vi "img test.vi"() -> ()   [LabVIEW 2009]
uses:
  <vilib>/vision/NI_Vision_Development_Module.lvlib
panel:
  in  "Operation 1":T1(ring)=enum."Erode"
  out "Image 4":T2(plugin-control)
  out "Image 3":T2(plugin-control)
  in  "Color Plane":i32(ring)=1 items=["Red", "Green", "Blue", "Hue", "Saturation", "Luminance", "Value", "Intensity"]
  in  "Structuring Element":i32[][](array[numeric])=[[1, 1, 1]]
  in  "startign rame":i32
  in  "Number of iterations (1)":i32=1
  in  "frame diff":i32
  out "Image 2":T2(plugin-control)
  in  "Range 2":cluster{"Lower value":sgl, "Upper value":sgl}={"Lower value"=128.0, "Upper value"=255.0} {"Upper value" format="%.2f"; "Lower value" format="%.2f"}
  in  "stop":bool
  in  "Range":cluster{"Lower value":sgl, "Upper value":sgl}={"Lower value"=128.0, "Upper value"=255.0} {"Upper value" format="%.2f"; "Lower value" format="%.2f"}
  out "Image":T2(plugin-control)
  in  "AVI Path":path=path "C:/Users/Kokum Weeratunga/Desktop/ChongWei vs LinDan (japan open 2010).avi"
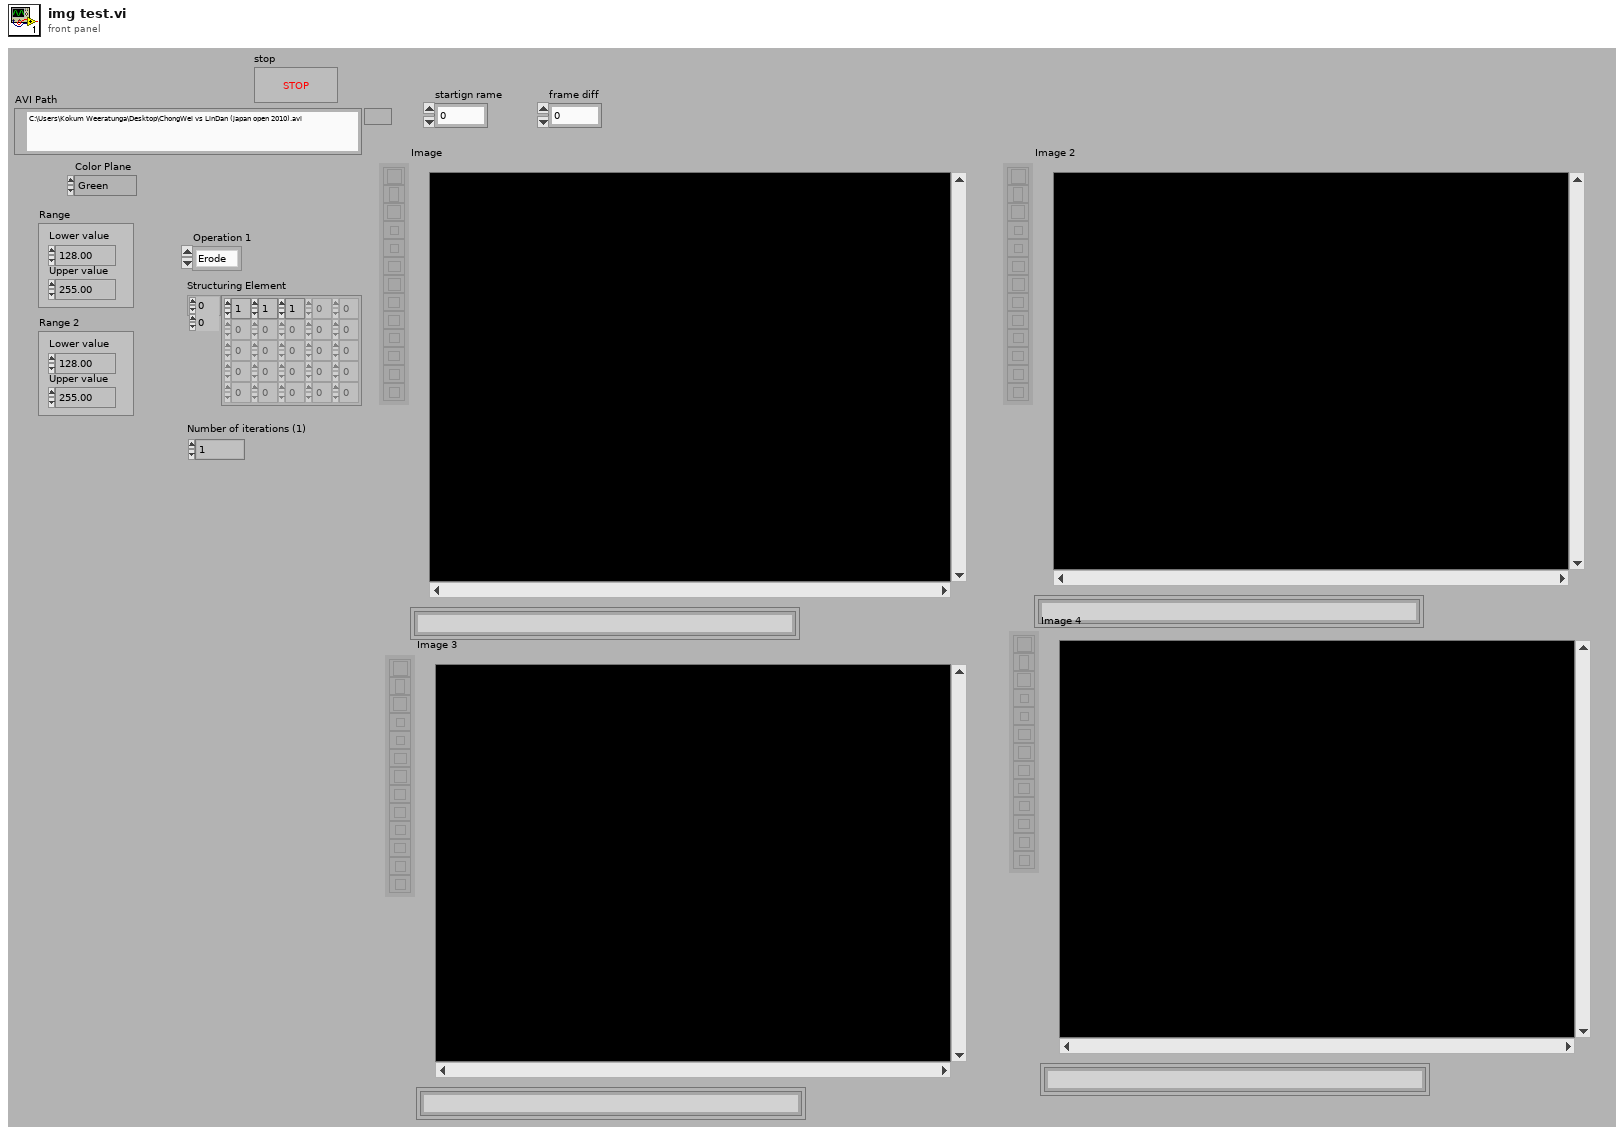
[diagram p1: front panel]
types:
  T1 = enum32{"AutoM", "Close", "Dilate", "Erode", "Gradient", "Gradient in", "Gradient out", "HitMiss", "Open", "PClose", "POpen", "Thick", "Thin"}
  T2 = typedef "IMAQ Image.ctl" = refnum<image>
  T3 = typedef "Image Type" = u32
  T4 = typedef "AviRefnum.ctl" = refnum<k1>
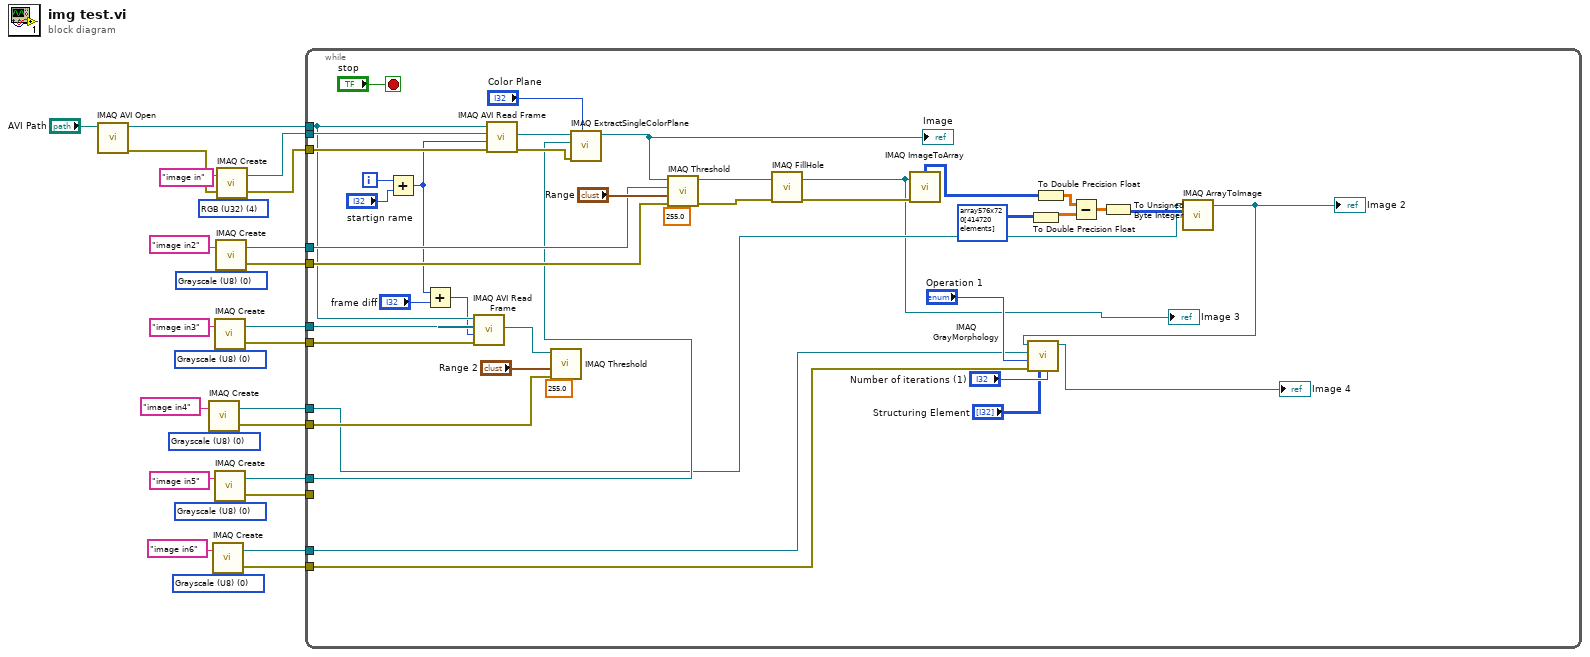
[diagram p0: block diagram]
diagram:
  w3 = T3 0 items=["Grayscale (U8)", "Grayscale (I16)", "Grayscale (SGL)", "Complex (CSG)", "RGB (U32)", "HSL (U32)", "RGB (U64)", "Grayscale (U16)"] ("Image Type")
  w14 = T3 0 items=["Grayscale (U8)", "Grayscale (I16)", "Grayscale (SGL)", "Complex (CSG)", "RGB (U32)", "HSL (U32)", "RGB (U64)", "Grayscale (U16)"] ("Image Type")
  w12 = T3 0 items=["Grayscale (U8)", "Grayscale (I16)", "Grayscale (SGL)", "Complex (CSG)", "RGB (U32)", "HSL (U32)", "RGB (U64)", "Grayscale (U16)"] ("Image Type")
  w16 = T3 0 items=["Grayscale (U8)", "Grayscale (I16)", "Grayscale (SGL)", "Complex (CSG)", "RGB (U32)", "HSL (U32)", "RGB (U64)", "Grayscale (U16)"] ("Image Type")
  w19 = T3 0 items=["Grayscale (U8)", "Grayscale (I16)", "Grayscale (SGL)", "Complex (CSG)", "RGB (U32)", "HSL (U32)", "RGB (U64)", "Grayscale (U16)"] ("Image Type")
  w22 = T3 4 items=["Grayscale (U8)", "Grayscale (I16)", "Grayscale (SGL)", "Complex (CSG)", "RGB (U32)", "HSL (U32)", "RGB (U64)", "Grayscale (U16)"] ("Image Type")
  n1 = call "IMAQ AVI Open"("AVI Path"="AVI Path") -> ("error out"=w26:errorcluster, "Avi Refnum"=w21:T4)  [unwired: 9 in]
  n2 = call "IMAQ Create"("Image Name"="image in4", "Image Type"=w14) -> ("New Image"=w8:T2, "error out"=w7:errorcluster)  [unwired: 3 in]
  n3 = call "IMAQ Create"("Image Name"="image in6", "Image Type"=w3) -> ("New Image"=w2:T2, "error out"=w1:errorcluster)  [unwired: 3 in]
  n4 = call "IMAQ Create"("Image Name"="image in3", "Image Type"=w12) -> ("New Image"=w10:T2, "error out"=w9:errorcluster)  [unwired: 3 in]
  n5 = call "IMAQ Create"("Image Name"="image in5", "Image Type"=w16) -> ("New Image"=w6:T2, "error out"=w5:errorcluster)  [unwired: 3 in]
  n6 = call "IMAQ Create"("Image Name"="image in2", "Image Type"=w19) -> ("New Image"=w18:T2, "error out"=w17:errorcluster)  [unwired: 3 in]
  n7 = call "IMAQ Create"("Image Name"="image in", "Image Type"=w22, "error in (no error)"=w26) -> ("New Image"=w23:T2, "error out"=w24:errorcluster)  [unwired: 2 in]
  n8 = while {
    tunnel: w24 -> [w69]
    tunnel: w23 -> [w68]
    tunnel: w21 -> [w59]
    tunnel: w18 -> [w65]
    tunnel: w17 -> [w64]
    tunnel: w10 -> [w58]
    tunnel: w9 -> [w57]
    tunnel: w8 -> [w33]
    tunnel: w7 -> [w42]
    tunnel: w6 -> [w43]
    tunnel: w5 -> [_]
    tunnel: w2 -> [w29]
    tunnel: w1 -> [w55]
    i -> [w52]
    stop <- "stop" stop-if-true
    n9 = Add(x=w52, y="startign rame") -> (x+y=w49:i32)
    n10 = Add(x=w49, y="frame diff") -> (x+y=w56:i32)
    n11 = call "IMAQ AVI Read Frame"("error in (no error)"=w57, "Frame Number"=w56, "Image"=w58, "Avi Refnum"=w59) -> ("Image Out"=w62:T2)  [unwired: 4 in, 3 out]
    n12 = call "IMAQ AVI Read Frame"("error in (no error)"=w69, "Frame Number"=w49, "Image"=w68, "Avi Refnum"=w59) -> ("error out"=w46:errorcluster, "Image Out"=w47:T2)  [unwired: 4 in, 2 out]
    n13 = call "IMAQ Threshold"("Replace Value"=sgl 255.0, "error in (no error)"=w42, "Range"="Range 2", "Image Src"=w62) -> ()  [unwired: 6 in, 2 out]
    n14 = call "IMAQ ExtractSingleColorPlane"("Color Plane"="Color Plane", "error in (no error)"=w46, "Image Dst"=w43, "Image Src"=w47) -> ("Image Dst Out"=w44:T2)  [unwired: 6 in, 1 out]
    "Image" <- w44
    n15 = call "IMAQ Threshold"("Replace Value"=sgl 255.0, "error in (no error)"=w64, "Range"="Range", "Image Dst"=w65, "Image Src"=w44) -> ("error out"=w40:errorcluster, "Image Dst Out"=w41:T2)  [unwired: 5 in]
    n16 = call "IMAQ FillHole"("error in (no error)"=w40, "Image Src"=w41) -> ("error out"=w36:errorcluster, "Image Dst Out"=w32:T2)  [unwired: 4 in]
    "Image 3" <- w32
    n17 = call "IMAQ ImageToArray"("error in (no error)"=w36, "Image"=w32) -> ("Image Pixels (U8)"=w35:u8[][])  [unwired: 2 in, 4 out]
    n18 = To Double Precision Float(number=u8[][] array576x720[414720 elements] ("Image Pixels (U8)")) -> (double precision float=w37:dbl[][])
    n19 = To Double Precision Float(number=w35) -> (double precision float=w38:dbl[][])
    n20 = Subtract(x=w38, y=w37) -> (x-y=w39:dbl[][])
    n21 = To Unsigned Byte Integer(number=w39) -> (unsigned 8bit integer=w34:u8[][])
    n22 = call "IMAQ ArrayToImage"("Image Pixels (U8)"=w34, "Image"=w33) -> ("Image Out"=w30:T2)  [unwired: 8 in, 1 out]
    "Image 2" <- w30
    n23 = call "IMAQ GrayMorphology"("Number of iterations (1)"="Number of iterations (1)", "Structuring Element"="Structuring Element", "error in (no error)"=w55, "Operation"="Operation 1", "Image Dst"=w29, "Image Src"=w30) -> ("Image Dst Out"=→"Image 4":T2)  [unwired: 4 in, 1 out]
  }
